vi "Read Manifold Valves.vi"(0 "Task In":refnum<k21>, 1 "Error In":errorcluster, 2 "Oxidizer":bool, 3 "Fuel":bool, 4 "Diluent":bool, 5 "Purge":bool, 6 "Vacuum":bool, 7 "Manifold Outlet":bool) -> (20 "Task Out":refnum<k21>, 21 "Error Out":errorcluster, 22 "Oxidizer State":bool, 23 "Fuel State":bool, 24 "Diluent State":bool, 25 "Purge State":bool, 26 "Vacuum State":bool, 27 "Manifold Outlet State":bool)   [LabVIEW 2018]
uses:
  <vilib>/DAQmx/write.llb/DAQmx Write (Digital 1D Bool 1Chan 1Samp).vi
  <vilib>/DAQmx/create/channels.llb/DAQmx Create Channel (DO-Digital Output).vi
  <vilib>/DAQmx/miscellaneous.llb/DAQmx Fill In Error Info.vi
panel:
  # "Valve Controls"
  # "TRUE:   valve open\nFALSE:  valve closed"
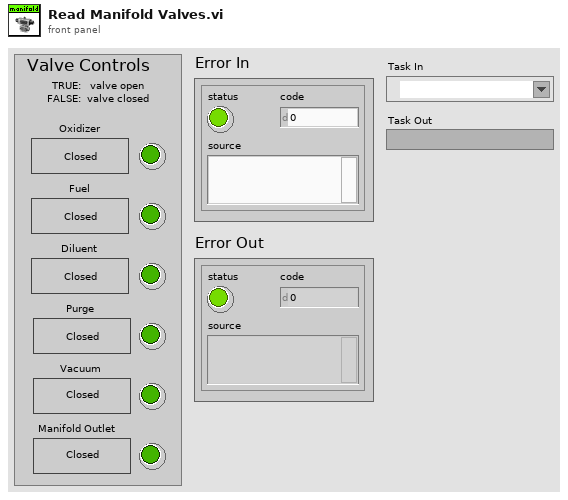
[diagram p1: front panel]
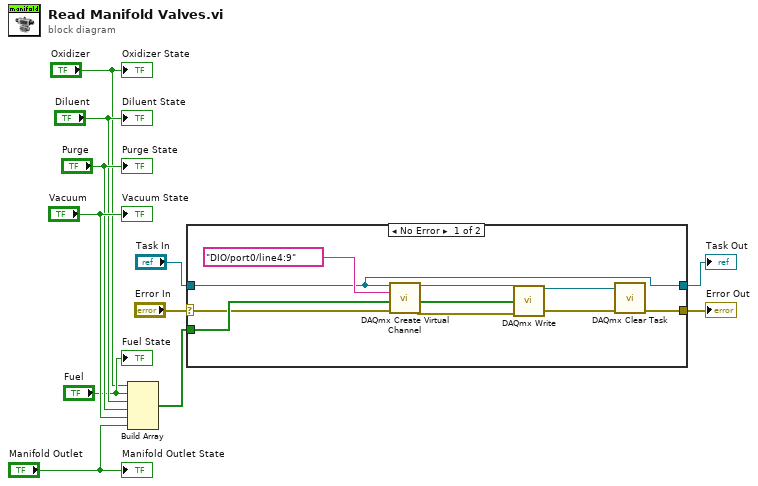
[diagram p0: block diagram]
diagram:
  n1 = Build Array("Oxidizer", "Fuel", "Diluent", "Purge", "Vacuum", "Manifold Outlet") -> (w9:bool[])
  n2 = case shown="No Error" "Error In" {
    selector: "Error In" -> [w12 w22]
    tunnel: [w18 w22] -> w10
    tunnel: w9 -> [w20 _]
    tunnel: "Task In" -> [w15 w21]
    tunnel: [w15 w21] -> w1
    frame No Error {
      n3 = call-poly <vilib>:"DAQmx Create Virtual Channel.vi"("task in"=w15, "lines"=tag "DIO/port0/line4:9", "error in"=w12) -> ("task out"=w17:refnum<k21>, "error out"=w13:errorcluster)  [unwired: 11 in]
      n4 = call-poly <vilib>:"DAQmx Write.vi"("task/channels in"=w17, "data"=w20, "error in"=w13) -> ("task out"=w16:refnum<k21>, "error out"=w14:errorcluster)  [unwired: 10 in, 1 out]
      n5 = call <vilib>:"DAQmx Clear Task.vi"("task in"=w16, "error in"=w14) -> ("error out"=w18:errorcluster)  [unwired: 13 in]
    }
    frame Error {
    }
  }
  "Error Out" <- w10
  "Task Out" <- w1
  "Oxidizer State" <- "Oxidizer"
  "Fuel State" <- "Fuel"
  "Diluent State" <- "Diluent"
  "Purge State" <- "Purge"
  "Vacuum State" <- "Vacuum"
  "Manifold Outlet State" <- "Manifold Outlet"
